vi "tlc_Play_Update Cue.vi"(8 "error in":errorcluster, 9 "Cue States":T1[][](array[typedef]), 10 "Cue Input":T2 {"Channels"."Intensity" min=0.0 max=100.0 step=1.0 format="%#.0f"}) -> (0 "error out":errorcluster, 2 "Cue Output":T2 {"Channels"."Intensity" min=0.0 max=100.0 step=1.0 format="%#.0f"})   [LabVIEW 2018]
doc: "This VI will increase or decrease the intensity of a channel in the Theatre Light Controller."
uses:
  Controls/tlc_Cue_Information.ctl
  Controls/channel.ctl
  Controls/Cue State.ctl
  Controls/tlc_User Interface Data Type.ctl
  Modules/Hardware/tlc_Hardware_Command Control.ctl
panel:
  # "Input"
  # "Output"
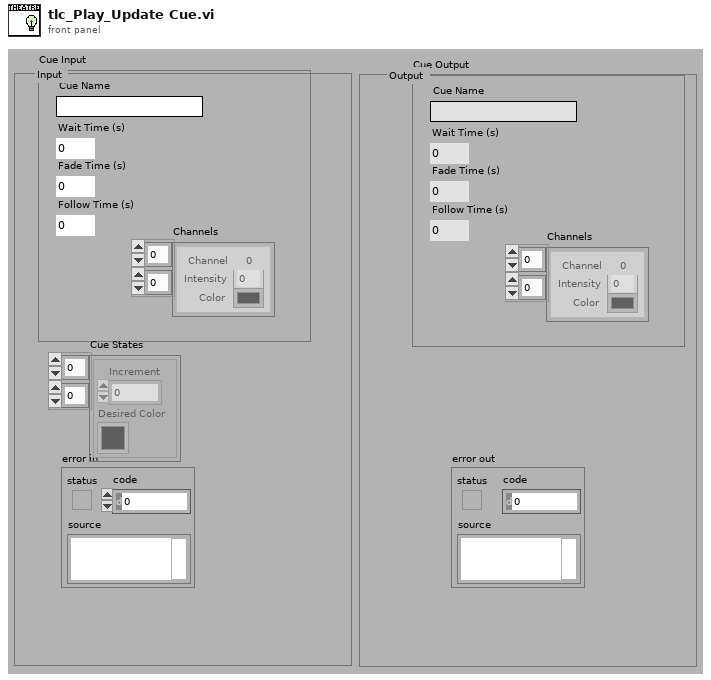
[diagram p1: front panel]
types:
  T1 = typedef "Cue State.ctl" = cluster{"Increment":dbl, "Desired Color":u32}
  T2 = typedef "tlc_Cue_Information.ctl" = cluster{"Cue Name":string, "Wait Time (s)":u32, "Fade Time (s)":u32, "Follow Time (s)":u32, "Channels":T3[][]}
  T3 = typedef "channel.ctl" = cluster{"Intensity":dbl, " Color":u32, "Channel":i32}
  T4 = typedef "tlc_User Interface Data Type.ctl" = enum16{"Initialize", "Initialize Front Panel", "Update Front Panel Channels", "Select Cue in Cue List", "Enable/Disable Front Panel Controls", "Update Cue List", "Stop"}
  T5 = typedef "tlc_Hardware_Command Control.ctl" = enum16{"Initialize", "Write", "Shutdown"}
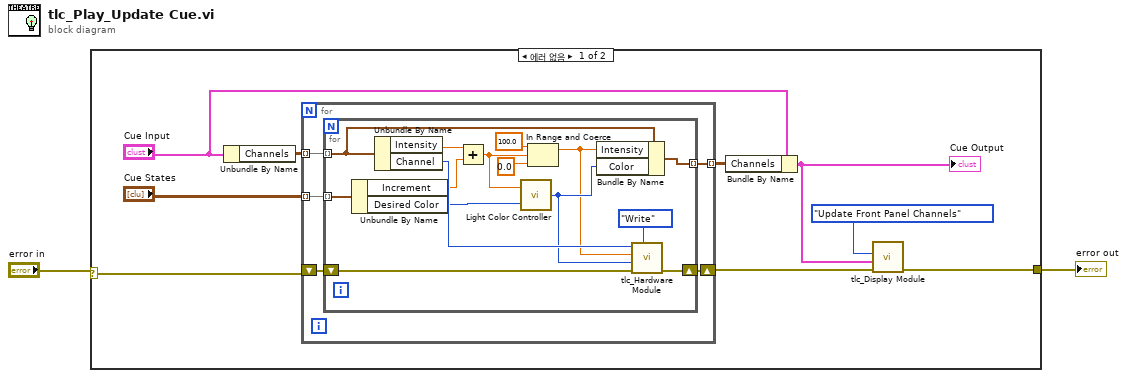
[diagram p0: block diagram]
diagram:
  n1 = case shown="에러 없음" "error in" {
    selector: "error in" -> [w4 w32]
    tunnel: [w3 w32] -> w1
    frame No Error {
      n2 = Unbundle By Name("Cue Input") -> ("Channels"=w10:T3[][])
      n3 = for {
        tunnel: w10 -> [w16] mode=indexing
        tunnel: [w15] -> w11 mode=indexing
        shift-right: [w13] -> w9
        shift-left: w4 -> [w14]
        tunnel: "Cue States" -> [w12] mode=indexing
        n4 = for {
          tunnel: w16 -> [w31] mode=indexing
          tunnel: [w30] -> w15 mode=indexing
          shift-right: [w27] -> w13
          shift-left: w14 -> [w28]
          tunnel: w12 -> [w25] mode=indexing
          n5 = Unbundle By Name(w25) -> ("Increment"=w23:dbl, "Desired Color"=w24:u32)
          n6 = Unbundle By Name(w31) -> ("Intensity"=w29:dbl, "Channel"=w26:i32)
          n7 = Add(x=w29, y=w23) -> (x+y=w20:dbl)
          n8 = call "Light Color Controller.vi"("Input Color"=w24, "Intensity"=w20) -> ("Output Color"=w21:u32)
          n9 = In Range and Coerce(upper limit=100.0, x=w20, lower limit=0.0) -> (coerced(x)=w17:dbl)  [unwired: 1 out]
          n10 = Bundle By Name(cluster=w31, "Intensity"=w17, "Color"=w21) -> (w30:T3)
          n11 = call "tlc_Hardware Module.vi"("Command (Write)"=tlc_Hardware_Command_Control."Write", "error in (no error)"=w28, "Color"=w21, "Intensity"=w17, "Channel"=w26) -> ("error out"=w27:errorcluster)  [unwired: 6 in]
        }
      }
      n12 = Bundle By Name(cluster="Cue Input", "Channels"=w11) -> (w6:T2)
      "Cue Output" <- w6
      n13 = call "tlc_Display Module.vi"("error in (no error)"=w9, "Data"=w6, "Data Type"=tlc_User_Interface_Data_Type."Update Front Panel Channels") -> ("error out"=w3:errorcluster)  [unwired: 8 in]
    }
    frame Error {
    }
  }
  "error out" <- w1
